vi "Load Tdm Wfm By Index.vi"(8 "error in (no error)":errorcluster, 10 "Read From":i32, 11 "file path":path) -> (0 "error out":errorcluster, 3 "Waveform":waveform(dbl)(graph))   [LabVIEW 2025, in "TDMS Waveform Creator UI.lvlib"]
uses:
  <vilib>/Platform/storage/lvStorage.llb/_openFunction.ctl
  <vilib>/Platform/storage/lvStorage.llb/_openStorageWithRootAutoDetect.vi
  <vilib>/Platform/storage/lvStorage.llb/xStorage/xStorageSupp/ErrorOut.vi
  <vilib>/Platform/storage/Storage.llb/__loadPropString.vi
  <vilib>/Platform/storage/Storage.llb/__loadPropTime.vi
  <vilib>/Platform/storage/Storage.llb/__loadPropRefList.vi
  <vilib>/Platform/storage/lvStorage.llb/_queryPropPoly.vi
  <vilib>/Platform/storage/lvStorage.llb/_queryPropString.vi
  <vilib>/Platform/storage/lvStorage.llb/_queryGenericObjects.vi
  <vilib>/Platform/storage/lvStorage.llb/_loadAllWaveform.vi
  <vilib>/Platform/storage/Storage.llb/Get Object Info.vi
  <vilib>/Platform/storage/Storage.llb/__closeStorageFromObject.vi
  <vilib>/Platform/storage/lvStorage.llb/xStorage/Open Data Storage/Open Data Storage.xnode
  <vilib>/Platform/storage/lvStorage.llb/xStorage/Get Properties/Get Properties.xnode
  <vilib>/Platform/storage/lvStorage.llb/xStorage/Read Data/Read Data.xnode
  <vilib>/Platform/storage/lvStorage.llb/xStorage/Close Data Storage/Close Data Storage.xnode
  TDMS Waveform Creator UI.lvlib
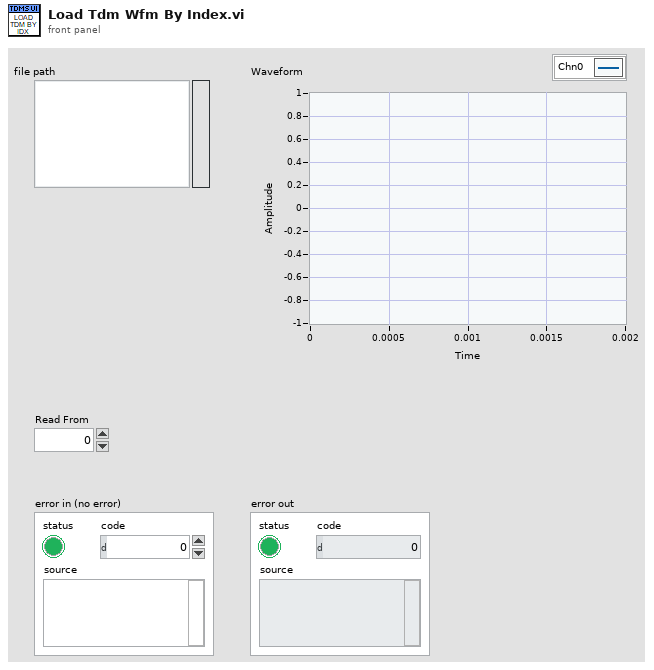
[diagram p1: front panel]
types:
  T1 = enum16{"UPDATE", "READ", "QUERY", "CREATE CHILD", "CREATE", "CONNECT", "DISCONNECT"}
  T2 = typedef "_openFunction.ctl" = enum16{"open", "open or create", "create or replace", "create", "open (read only)"}
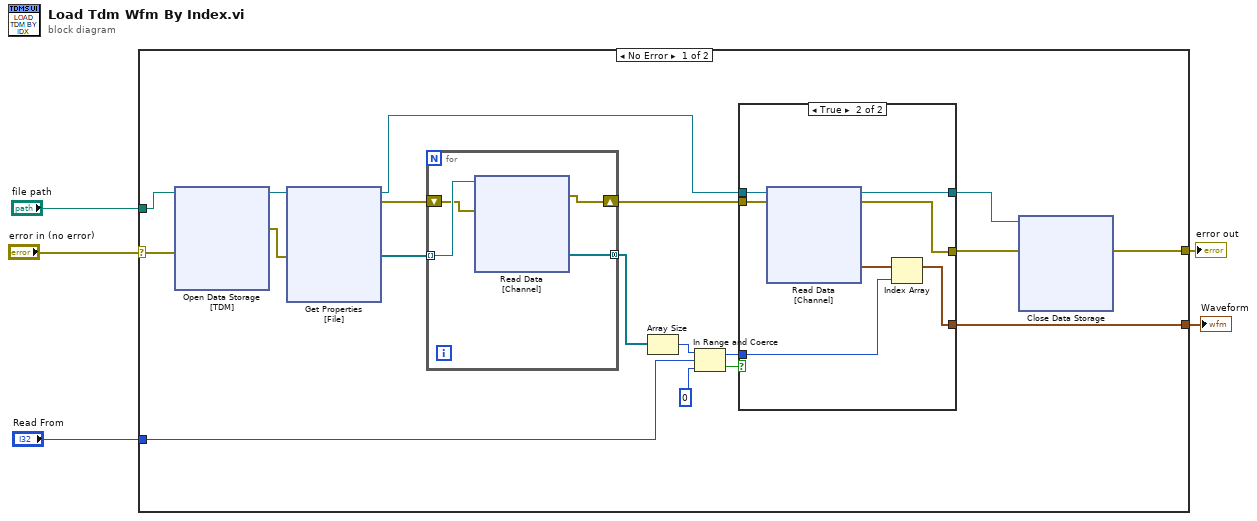
[diagram p0: block diagram]
diagram:
  n1 = case shown="No Error" "error in (no error)" {
    selector: "error in (no error)" -> [w19 w111]
    tunnel: "file path" -> [w10 _]
    tunnel: [w23 _] -> w4
    tunnel: "Read From" -> [w20 _]
    tunnel: [w11 w111] -> w1
    frame No Error {
      n2 = xnode "Open Data Storage\n[TDM]"("file path"=w10, "error in (no error)"=w19) -> ("storage refnum (file)"=w9:refnum<k20>, "error out"=w16:errorcluster)  [unwired: 3 in, 1 out]
      n3 = xnode "Get Properties\n[File]"("storage refnum (file)"=w9, "error in"=w16) -> ("storage refnum (file) out"=w7:refnum<k20>, "error out"=w15:errorcluster, "storage refnums (channel group)"=w18:refnum<k20>[])  [unwired: 5 out]
      n4 = for {
        tunnel: w18 -> [w60] mode=indexing
        tunnel: [w59] -> w14 mode=concatenating
        shift-right: [w57] -> w13
        shift-left: w15 -> [w58]
        n5 = xnode "Read Data\n[Channel]"("storage refnum (channel group)"=w60, "error in"=w58) -> ("storage refnums (channel)"=w59:refnum<k20>[], "error out"=w57:errorcluster)  [unwired: 1 out]
      }
      n6 = Array Size(array=w14) -> (size(s)=w22:i32)
      n7 = In Range and Coerce(upper limit=w22, x=w20, lower limit=0) -> (coerced(x)=w8:i32, In Range?=w17:bool)
      n8 = case shown="True" w17 {
        tunnel: [w33 w40] -> w12
        tunnel: [_ w37] -> w23
        tunnel: w13 -> [w33 w39]
        tunnel: w8 -> [_ w36]
        tunnel: w7 -> [w32 w35]
        tunnel: [w32 w34] -> w6
        frame False {
        }
        frame True {
          n9 = xnode "Read Data\n[Channel]"("storage refnum (file)"=w35, "error in"=w39) -> ("Signal"=w38:waveform(dbl)[], "storage refnum (file) out"=w34:refnum<k20>, "error out"=w40:errorcluster)  [unwired: 2 in, 1 out]
          n10 = Index Array(array=w38, index=w36) -> (element=w37:waveform(dbl))
        }
      }
      n11 = xnode "Close Data Storage\n"("storage refnum (file)"=w6, "error in (no error)"=w12) -> ("error out"=w11:errorcluster)  [unwired: 1 out]
    }
    frame Error {
    }
  }
  "Waveform" <- w4
  "error out" <- w1
